vi "ReadSubVI.vi"(2 "reference":refnum<vi>) -> (1 "SubVI":T6)   [LabVIEW 2013]
uses:
  <vilib>/Utility/miscctls.llb/LVBoundsTypeDef.ctl
  <vilib>/Utility/miscctls.llb/LVRectTypeDef.ctl
  <vilib>/Utility/miscctls.llb/LVPositionTypeDef.ctl
  <vilib>/Utility/miscctls.llb/LVBreakpointStatusEnum.ctl
  <vilib>/picture/picture.llb/imagedata.ctl
panel:
  out "error out":errorcluster
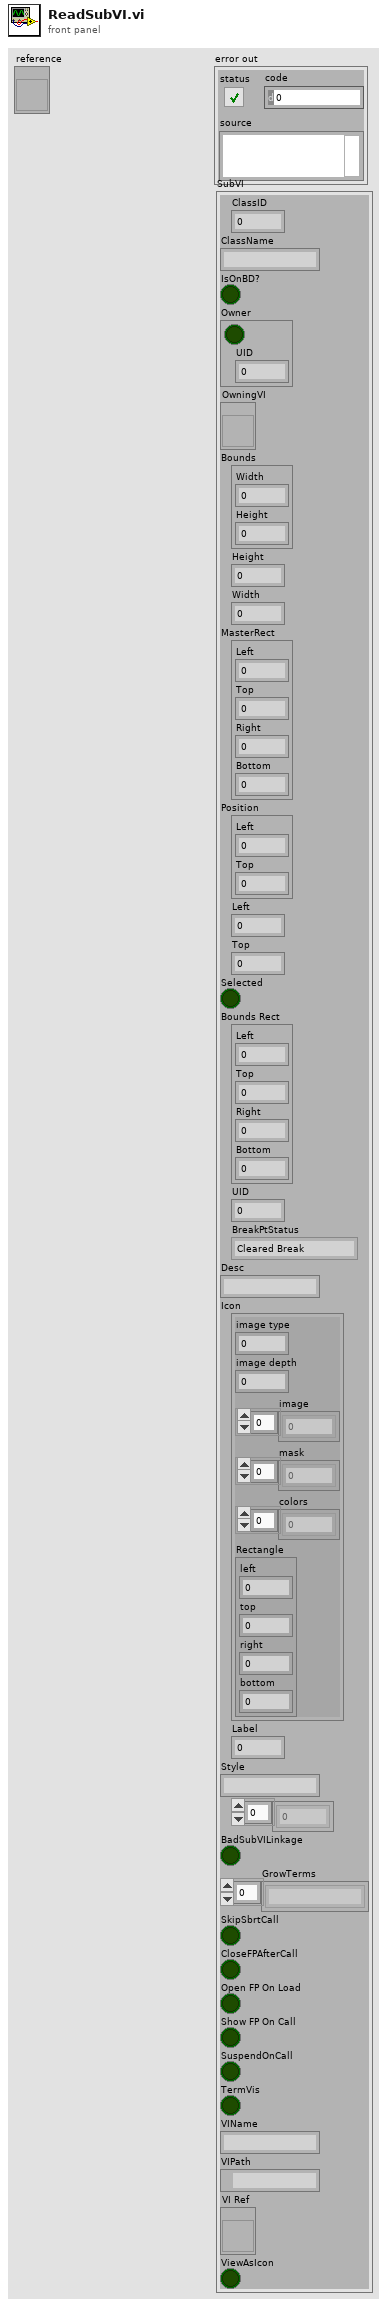
[diagram p1: front panel]
types:
  T1 = typedef "LVBoundsTypeDef.ctl" = cluster{"Width":u32, "Height":u32}
  T2 = typedef "LVRectTypeDef.ctl" = cluster{"Left":i16, "Top":i16, "Right":i16, "Bottom":i16}
  T3 = typedef "LVPositionTypeDef.ctl" = cluster{"Left":i32, "Top":i32}
  T4 = typedef "LVBreakpointStatusEnum.ctl" = enum8{"Cleared Break", "Enabled Break", "Disabled Break"}
  T5 = typedef "imagedata.ctl" = cluster{"image type":i32, "image depth":i32, "image":u8[], "mask":u8[], "colors":u32[], "Rectangle":cluster{"left":i16, "top":i16, "right":i16, "bottom":i16}}
  T6 = cluster{"ClassID":u32, "ClassName":string, "IsOnBD?":bool, "Owner":cluster{bool, "UID":i32}, "OwningVI":refnum<vi>, "Bounds":T1, "Height":u32, "Width":u32, "MasterRect":T2, "Position":T3, "Left":i32, "Top":i32, "Selected":bool, "Bounds Rect":T2, "UID":i32, "BreakPtStatus":T4, "Desc":string, "Icon":T5, "Label":i32, "Style":string, "Terms[]":i32[], "BadSubVILinkage":bool, "GrowTerms":string[], "SkipSbrtCall":bool, "CloseFPAfterCall":bool, "Open FP On Load":bool, "Show FP On Call":bool, "SuspendOnCall":bool, "TermVis":bool, "VIName":string, "VIPath":path, "VI Ref":refnum<vi>, "ViewAsIcon":bool}
  T7 = cluster{"ClassID":u32, "ClassName":string, "IsOnBD?":bool, "Cluster":cluster{bool, "UID":i32}, "OwningVI":refnum<vi>, "Bounds":T1, "Height":u32, "Width":u32, "MasterRect":T2, "Position":T3, "Left":i32, "Top":i32, "Selected":bool, "Bounds Rect":T2, "UID":i32, "BreakPtStatus":T4, "Desc":string, "Icon":T5, "UID":i32, "Style":string, i32[], "BadSubVILinkage":bool, "GrowTerms":string[], "SkipSbrtCall":bool, "CloseFPAfterCall":bool, "Open FP On Load":bool, "Show FP On Call":bool, "SuspendOnCall":bool, "TermVis":bool, "VIName":string, "VIPath":path, "VI Ref":refnum<vi>, "ViewAsIcon":bool}
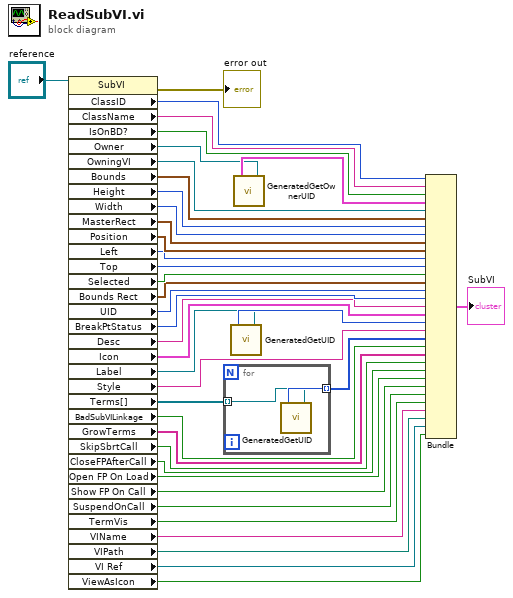
[diagram p0: block diagram]
diagram:
  n1 = property class="SubVI"(reference="reference") -> (error out=→"error out":errorcluster, "ClassID"=w38:u32, "ClassName"=w37:string, "IsOnBD?"=w36:bool, "Owner"=w34:refnum<vi>, "OwningVI"=w33:refnum<vi>, "Bounds"=w32:T1, "Height"=w31:u32, "Width"=w30:u32, "MasterRect"=w29:T2, "Position"=w28:T3, "Left"=w27:i32, "Top"=w26:i32, "Selected"=w25:bool, "Bounds Rect"=w24:T2, "UID"=w23:i32, "BreakPtStatus"=w22:T4, "Desc"=w21:string, "Icon"=w20:T5, "Label"=w18:refnum<vi>, "Style"=w17:string, "Terms[]"=w15:refnum<vi>[], "BadSubVILinkage"=w14:bool, "GrowTerms"=w13:string[], "SkipSbrtCall"=w12:bool, "CloseFPAfterCall"=w11:bool, "Open FP On Load"=w10:bool, "Show FP On Call"=w9:bool, "SuspendOnCall"=w8:bool, "TermVis"=w7:bool, "VIName"=w6:string, "VIPath"=w5:path, "VI Ref"=w4:refnum<vi>, "ViewAsIcon"=w3:bool)  [unwired: 1 in, 1 out]
  n2 = for {
    tunnel: [w41] -> w16 mode=indexing
    tunnel: w15 -> [w40] mode=indexing
    n3 = call "GeneratedGetUID.vi"("Text in"=w40) -> ("UID"=w41:i32)
  }
  n4 = call "GeneratedGetUID.vi"("Text in"=w18) -> ("UID"=w19:i32)
  n5 = call "GeneratedGetOwnerUID.vi"("Generic in"=w34) -> ("Cluster"=w35:cluster{bool, "UID":i32})
  n6 = Bundle("ClassID"=w38, "ClassName"=w37, "IsOnBD?"=w36, "Cluster"=w35, "OwningVI"=w33, "Bounds"=w32, "Height"=w31, "Width"=w30, "MasterRect"=w29, "Position"=w28, "Left"=w27, "Top"=w26, "Selected"=w25, "Bounds Rect"=w24, "UID"=w23, "BreakPtStatus"=w22, "Desc"=w21, "Icon"=w20, "UID"=w19, "Style"=w17, w16, "BadSubVILinkage"=w14, "GrowTerms"=w13, "SkipSbrtCall"=w12, "CloseFPAfterCall"=w11, "Open FP On Load"=w10, "Show FP On Call"=w9, "SuspendOnCall"=w8, "TermVis"=w7, "VIName"=w6, "VIPath"=w5, "VI Ref"=w4, "ViewAsIcon"=w3) -> (→"SubVI":T7)  [unwired: 1 in]
